vi "Position Check.vi"(8 "data value reference 2":refnum<data-value>, 11 "data value reference":refnum<data-value>) -> (0 "Y-Offset":dbl, 1 "X-Offset":dbl, 2 "XY Graph":T1(graph))   [LabVIEW 2021]
uses:
  State Estimator/Measurements.ctl
  IMU/IMU Data.ctl
  Steering Motor Encoder/Steering Motor Encoder Data.ctl
  GNSS/GNSS Data.ctl
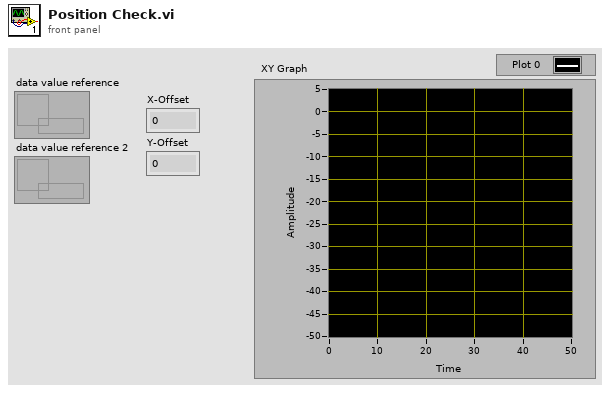
[diagram p1: front panel]
types:
  T1 = cluster{"Trajectory(X/Y/PSI)":dbl[], "Trajectory(X/Y/PSI)":dbl[]}
  T2 = typedef "Measurements.ctl" = cluster{"IMU Data":T3, "Steering Motor Encoder Data":T4, "GNSS Data":T5}
  T3 = typedef "IMU Data.ctl" = cluster{"Gyroscope":cluster{"X (rad/s)":dbl, "Y (rad/s)":dbl, "Z (rad/s)":dbl}, "Accelerometer":cluster{"X (m/s^2)":dbl, "Y (m/s^2)":dbl, "Z (m/s^2)":dbl}, "Flag IMU":dbl}
  T4 = typedef "Steering Motor Encoder Data.ctl" = cluster{"Encoder Position (counts)":i32, "Steering Angle (rad)":dbl, "Flag Steering Encoder":dbl}
  T5 = typedef "GNSS Data.ctl" = cluster{"Latitude (rad)":dbl, "Longitude (rad)":dbl, "Altitude (m)":dbl, "Speed (m/s)":dbl, "Heading (rad)":dbl, "Fix Quality":i32, "Number of Satellites":i32, "Latitude (deg)":dbl, "Longitude (deg)":dbl, "Flag GNSS":dbl}
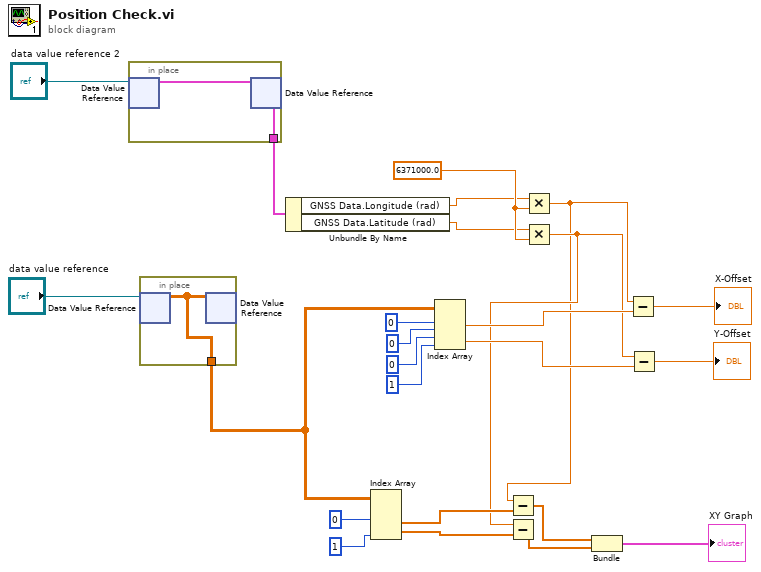
[diagram p0: block diagram]
diagram:
  w7 = 6371000.0
  n1 = in-place {
    in-place-border: [w25] -> w20
    n2 = in-place-dvr #1("data value reference 2") -> (w25:T2)  [unwired: 1 out]
    n3 = in-place-dvr #1(w25) -> ()  [unwired: 2 out]
  }
  n4 = in-place {
    in-place-border: [w26] -> w15
    n5 = in-place-dvr #2("data value reference") -> (w26:dbl[][])  [unwired: 1 out]
    n6 = in-place-dvr #2(w26) -> ()  [unwired: 2 out]
  }
  n7 = Unbundle By Name(w20) -> ("GNSS Data.Longitude (rad)"=w6:dbl, "GNSS Data.Latitude (rad)"=w5:dbl)
  n8 = Index Array(array=w15, index (col) #1=0, index (col) #2=1) -> (element #1=w12:dbl[], element #2=w11:dbl[])  [unwired: 2 in]
  n9 = Index Array(array=w15, index (row) #1=0, index (col) #1=0, index (row) #2=0, index (col) #2=1) -> (element #1=w4:dbl, element #2=w3:dbl)
  n10 = Multiply(x=w6, y=w7) -> (x*y=w1:dbl)
  n11 = Subtract(x=w1, y=w12) -> (x-y=w10:dbl[])
  n12 = Multiply(x=w5, y=w7) -> (x*y=w2:dbl)
  n13 = Subtract(x=w2, y=w11) -> (x-y=w9:dbl[])
  n14 = Bundle(w10, w9) -> (→"XY Graph":cluster{dbl[], dbl[]})  [unwired: 1 in]
  n15 = Subtract(x=w1, y=w4) -> (x-y=→"X-Offset":dbl)
  n16 = Subtract(x=w2, y=w3) -> (x-y=→"Y-Offset":dbl)
